vi "Pixellate.vi"(8 "error in":errorcluster, 11 "BigMAQ in":refnum<class "BigMAQ.lvclass">) -> (0 "error out":errorcluster, 3 "BigMAQ out":refnum<class "BigMAQ.lvclass">)   [LabVIEW 2019, in "BigMAQ.lvclass"]
uses:
  BigMAQ.lvclass
  BigMAQ.lvclass/BigMAQ.ctl
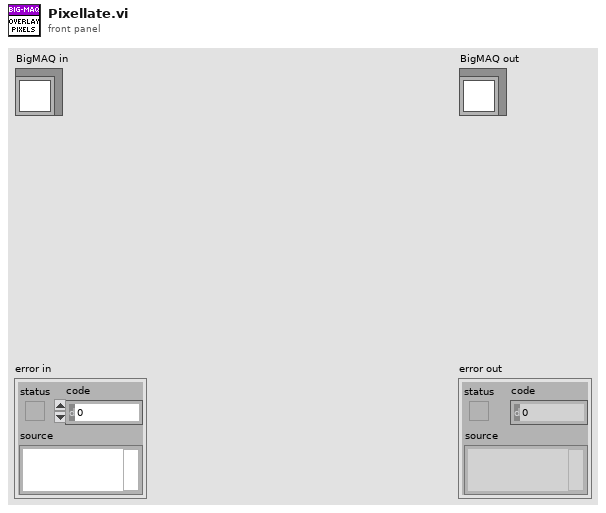
[diagram p1: front panel]
types:
  T1 = typedef "BigMAQ.lvclass/Overlay.ctl" = cluster{"Name":string, "Data":cluster{"Points":cluster{"X":dbl, "Y":dbl}[], "Voltages":dbl[]}}
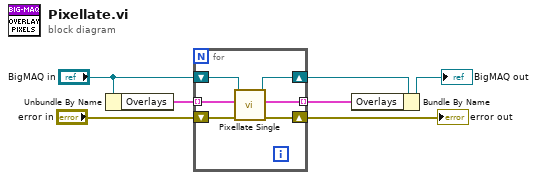
[diagram p0: block diagram]
diagram:
  n1 = Unbundle By Name("BigMAQ in") -> ("Overlays"=w7:T1[])
  n2 = for {
    tunnel: w7 -> [w12] mode=indexing
    tunnel: [w13] -> w5 mode=indexing
    shift-right: [w9] -> w3
    shift-left: "BigMAQ in" -> [w8]
    shift-right: [w10] -> w1
    shift-left: "error in" -> [w11]
    n3 = call "Pixellate Single.vi"("error in"=w11, "Overlay"=w12, "BigMAQ in"=w8) -> ("error out"=w10:errorcluster, "Pixellated Overlay"=w13:T1, "BigMAQ out"=w9:refnum<class "BigMAQ.lvclass">)  [unwired: 6 in]
  }
  "error out" <- w1
  n4 = Bundle By Name(cluster=w3, "Overlays"=w5) -> (→"BigMAQ out":refnum<class "BigMAQ.lvclass">)
